vi "Read log.vi"(8 "error in (no error)":errorcluster, 11 "Instr Actor in":refnum<class "Instr Actor.lvclass">) -> (0 "error out":errorcluster, 2 "Session Handle":T1, 3 "Instr Actor out":refnum<class "Instr Actor.lvclass">)   [LabVIEW 2014, in "Instrument Library.lvlib" / "Instr Actor.lvclass"]
uses:
  Instr Actor.lvclass
  <userlib>/_Session Fwk/Typedefs/Session Handle.ctl
  <userlib>/_Session Fwk/Session - Root.lvclass
  Instr Actor.lvclass/Instr Actor.ctl
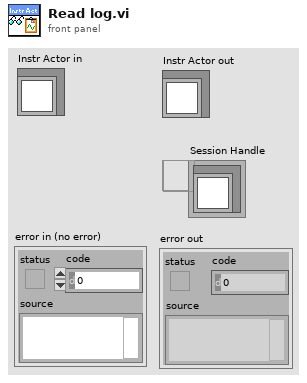
[diagram p1: front panel]
types:
  T1 = typedef "Session - Root.lvclass/Session Handle.ctl" = refnum<data-value>
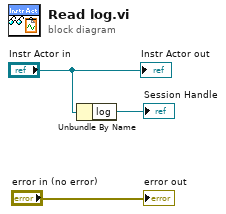
[diagram p0: block diagram]
diagram:
  n1 = Unbundle By Name("Instr Actor in") -> ("log"=→"Session Handle":T1)
  "error out" <- "error in (no error)"
  "Instr Actor out" <- "Instr Actor in"
